vi "Write Ghosts.vi"(8 "error in (no error)":errorcluster, 10 "Ghosts":T1, 11 "Ghosts in":refnum<class "Ghosts.lvclass">) -> (0 "error out":errorcluster, 3 "Ghosts out":refnum<class "Ghosts.lvclass">)   [LabVIEW 2016, in "PacManClasses.lvlib" / "Ghosts.lvclass"]
uses:
  Ghosts.lvclass
  Generic Controls/Ghosts.ctl
  Ghosts.lvclass/Ghosts.ctl
  PacManClasses.lvlib
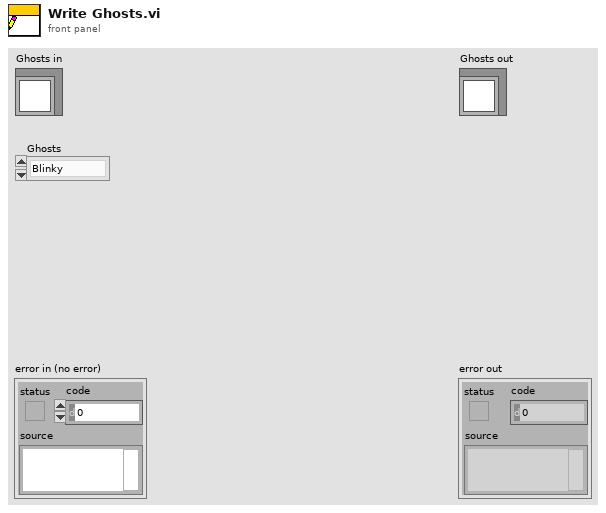
[diagram p1: front panel]
types:
  T1 = typedef "PacManClasses.lvlib/Ghosts.ctl" = enum16{"Blinky", "Pinky", "Inky", "Clyde"}
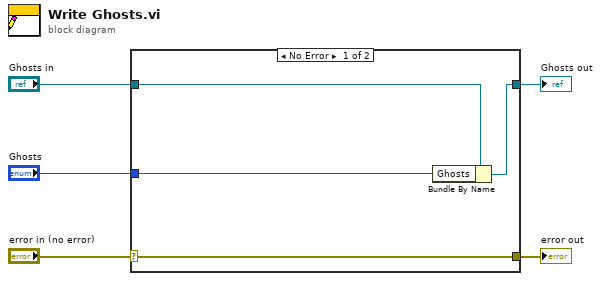
[diagram p0: block diagram]
diagram:
  n1 = case shown="No Error" "error in (no error)" {
    selector: "error in (no error)" -> [w9 w10]
    tunnel: [w9 w10] -> w4
    tunnel: [w7 w11] -> w2
    tunnel: "Ghosts in" -> [w8 w11]
    tunnel: "Ghosts" -> [w6 _]
    frame No Error {
      n2 = Bundle By Name(cluster=w8, "Ghosts"=w6) -> (w7:refnum<class "Ghosts.lvclass">)
    }
    frame Error {
    }
  }
  "error out" <- w4
  "Ghosts out" <- w2
